vi "Read Timeout (1s).vi"(8 "error in (no error)":errorcluster, 11 "MiniIO in":refnum<class "MiniIO.lvclass">) -> (0 "error out":errorcluster, 2 "Timeout (1s)":i32=1000, 3 "MiniIO out":refnum<class "MiniIO.lvclass">)   [LabVIEW 2018, in "MiniIO.lvlib" / "MiniIO.lvclass"]
uses:
  MiniIO.lvclass
  MiniIO.lvclass/MiniIO.ctl
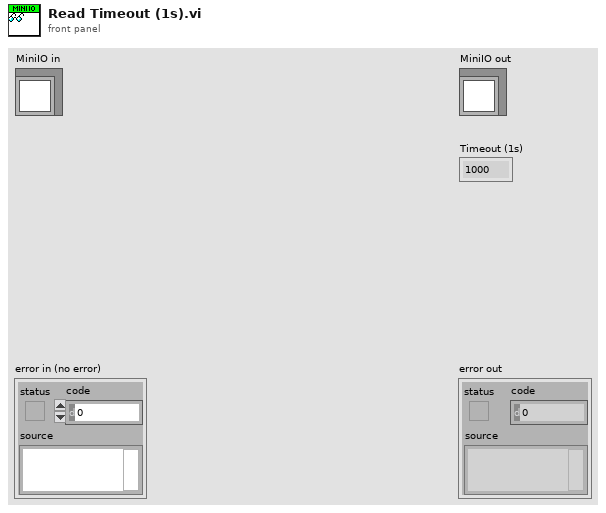
[diagram p1: front panel]
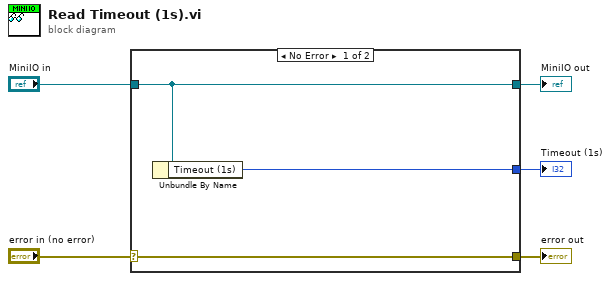
[diagram p0: block diagram]
diagram:
  n1 = case shown="No Error" "error in (no error)" {
    selector: "error in (no error)" -> [w8 w9]
    tunnel: [w8 w9] -> w4
    tunnel: [w7 w10] -> w2
    tunnel: "MiniIO in" -> [w7 w10]
    tunnel: [w6 _] -> w1
    frame No Error {
      n2 = Unbundle By Name(w7) -> ("Timeout (1s)"=w6:i32)
    }
    frame Error {
    }
  }
  "error out" <- w4
  "MiniIO out" <- w2
  "Timeout (1s)" <- w1
